vi "Get Size of Data from TD - Variant Error Cluster - Returns Correct Size.vi"() -> ()   [LabVIEW 2017, in "Composition.Tests.lvlib"]
uses:
  Composition.Tests.lvlib
  <vilib>/addons/_JKI Toolkits/Caraya/classes/Assert/Assert Equal Value_Variant.vi
  Composition/Composition.lvlib
  <vilib>/addons/_JKI Toolkits/Caraya/classes/Test/Test.lvclass
  <vilib>/addons/_JKI Toolkits/Caraya/classes/Assert/Assert.lvclass
panel:
  out "error out":errorcluster
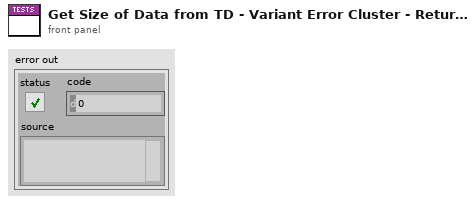
[diagram p1: front panel]
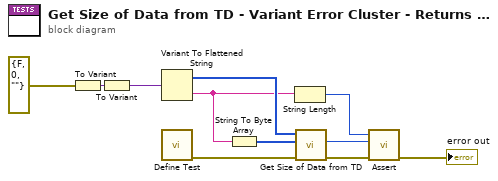
[diagram p0: block diagram]
diagram:
  n1 = To Variant(anything=errorcluster {"status"=FALSE, "code"=0, "source"=""}) -> (Variant=w11:variant)
  n2 = To Variant(anything=w11) -> (Variant=w9:variant)
  n3 = Variant To Flattened String(Variant=w9) -> (data string=w2:string, 1:w3:i16[])
  n4 = call <vilib>:"Define Test.vi"() -> ("error out"=w8:errorcluster)  [unwired: 10 in, 1 out]
  n5 = String To Byte Array(string=w2) -> (unsigned byte array=w10:u8[])
  n6 = String Length(string=w2) -> (length=w4:i32)
  n7 = call "Get Size of Data from TD.vi"("error in (no error)"=w8, "Data String"=w10, "Type Descriptor"=w3) -> ("error out"=w7:errorcluster, "Size of Data"=w6:i32)  [unwired: 7 in]
  n8 = call-poly <vilib>:"Assert.vi"("error in (no error)"=w7, "Y"=w6, "X"=w4) -> ("error out"=→"error out":errorcluster)  [unwired: 7 in, 1 out]
